vi "AddWindowInstance.vi"(8 "error in (no error)":errorcluster, 9 "Window Instance":refnum<class "Window.lvclass">, 10 "SDL_Window *":i64, 11 "Engine in":refnum<class "Engine.lvclass">) -> (0 "error out":errorcluster, 3 "Engine out":refnum<class "Engine.lvclass">)   [LabVIEW 2024, in "GLF.lvlib" / "Engine.lvclass"]
uses:
  Engine.lvclass
  Engine.lvclass/Engine.ctl
  Window/Window.lvclass
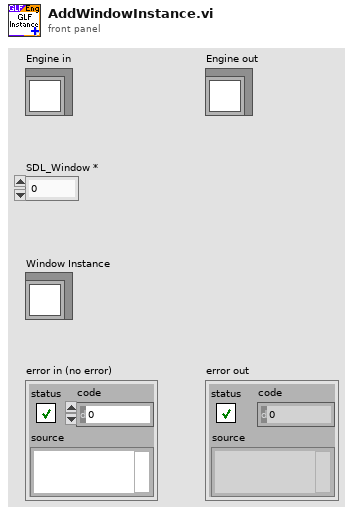
[diagram p1: front panel]
types:
  T1 = typedef "GLF.lvlib/Engine.lvclass/DVR--cluster.ctl" = cluster{"CMD Queue":T2, "Config":T3, "Ctxt":T5, "Metrics":T6, "GLF Instances":set{refnum<class "IAmGLF.lvclass">}, "Window Instances":map{i64, refnum<class "Window.lvclass">}}
  T2 = typedef "GLF.lvlib/Engine.lvclass/Command--queue.ctl" = refnum<queue>
  T3 = typedef "GLF.lvlib/Engine.lvclass/Config--cluster.ctl" = cluster{"Quit On Last Window Closed":bool, "VSync":T4, "FPS Target":dbl}
  T4 = typedef "GLF.lvlib/Engine.lvclass/VSync--enum.ctl" = enum16{"Disabled", "Enabled", "Adaptative"}
  T5 = typedef "GLF.lvlib/Engine.lvclass/Context--cluster.ctl" = cluster{"Ticks Begin":u64, "VSync Enabled":bool}
  T6 = typedef "GLF.lvlib/Engine.lvclass/Metrics--cluster.ctl" = cluster{"Uptime [ms]":u64, "Loop Time [ms]":u64}
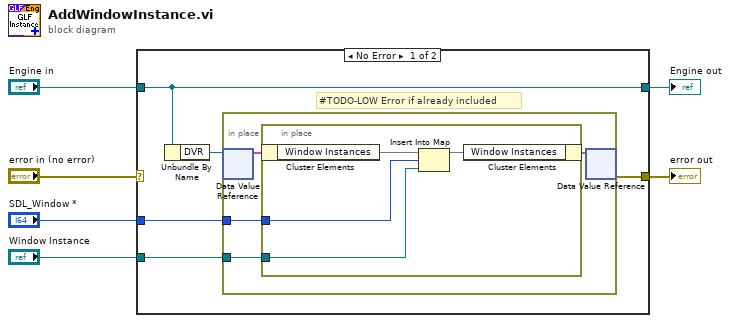
[diagram p0: block diagram]
diagram:
  n1 = case shown="No Error" "error in (no error)" {
    selector: "error in (no error)" -> [_ w21]
    tunnel: [w9 w21] -> w5
    tunnel: [w11 w20] -> w3
    tunnel: "Engine in" -> [w11 w20]
    tunnel: "Window Instance" -> [w8 _]
    tunnel: "SDL_Window *" -> [w7 _]
    frame No Error {
      # "#TODO-LOW Error if already included"
      n2 = Unbundle By Name(w11) -> ("DVR"=w10:refnum<data-value>)
      n3 = in-place {
        in-place-border: w8 -> [w13]
        in-place-border: w7 -> [w12]
        n4 = in-place-dvr #1(w10) -> (w15:T1)  [unwired: 1 out]
        n5 = in-place {
          in-place-border: w13 -> [w16]
          in-place-border: w12 -> [w17]
          n6 = in-place-cluster #2(w15) -> ("Window Instances"=w19:map{i64, refnum<class "Window.lvclass">})
          n7 = Insert Into Map(map in=w19, key=w17, value=w16) -> (map out=w18:map{i64, refnum<class "Window.lvclass">})  [unwired: 2 out]
          n8 = in-place-cluster #2("Window Instances"=w18) -> (w14:T1)
        }
        n9 = in-place-dvr #1(w14) -> (w9:errorcluster)  [unwired: 1 out]
      }
    }
    frame Error {
    }
  }
  "error out" <- w5
  "Engine out" <- w3
